vi "Datalog append DATA, Mode 1.vi"(0 "Datalog (Data) path":path=path "C:/test/test_D.log", 2 "Data (Mode 1)":T1[](array[typedef]), 3 "Error in":errorcluster) -> (6 "Path out":path, 9 "Error out":errorcluster)   [LabVIEW 2015]
uses:
  Ctls/Data values, Mode 1 (for datalog).ctl
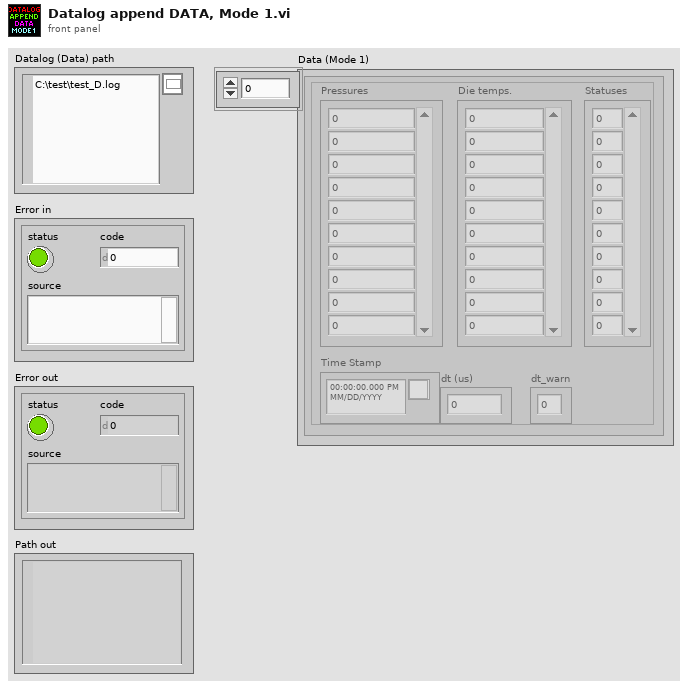
[diagram p1: front panel]
types:
  T1 = typedef "Data values, Mode 1 (for datalog).ctl" = cluster{"Time Stamp":timestamp, "dt (us)":sgl, "dt_warn":u8, "Pressures":sgl[], "Die temps.":sgl[], "Statuses":u8[]}
  T2 = enum16{"open", "replace", "create", "open or create", "replace or create", "replace or create with confirmation"}
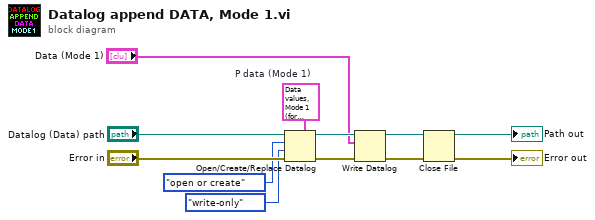
[diagram p0: block diagram]
diagram:
  w1 = T1 {"Time Stamp"=timestamp(0 s since 1904-01-01), "dt (us)"=0.0, "dt_warn"=0, "Pressures"=[], "Die temps."=[], "Statuses"=[]}  # P data (Mode 1)
  n1 = Open/Create/Replace Datalog(5:w1, 8:"Error in", 9:enum16{"read/write", "read-only", "write-only"}."write-only" ("access (0:read/write)"), 10:T2."open or create" ("operation (0:open)"), 11:"Datalog (Data) path") -> (0:w8:errorcluster, 3:w7:refnum<k1>)  [unwired: 1 in, 1 out]
  n2 = Write Datalog(4:w8, 6:"Data (Mode 1)", 7:w7) -> (0:w6:errorcluster, 3:w5:refnum<k1>)
  n3 = Close File(refnum=w5, error in=w6) -> (path=→"Path out":path, error out=→"Error out":errorcluster)
